vi "Get Data From Binary Block.vi"(10 "Binary Block":string) -> (2 "Data Part":string)   [LabVIEW 2016, in "Agilent 3352X Series.lvlib"]
doc: "For an IEEE Binary Block of values of the format #<n><n_digits><data>, get the <data> part of it"
uses:
  Agilent 3352X Series.lvlib
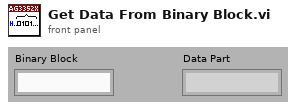
[diagram p1: front panel]
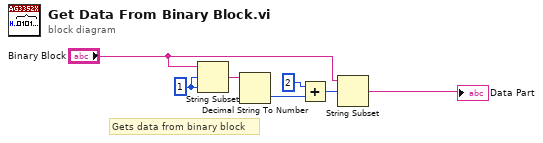
[diagram p0: block diagram]
diagram:
  w1 = 1 ("length (rest)")
  # "Gets data from binary block"
  n1 = String Subset(string="Binary Block", offset (0)=w1, length (rest)=w1) -> (substring=w7:string)
  n2 = Decimal String To Number(string=w7) -> (number=w4:i32)  [unwired: 3 out]
  n3 = Add(x=2 ("offset (0)"), y=w4) -> (x+y=w5:i32)
  n4 = String Subset(string="Binary Block", offset (0)=w5) -> (substring=→"Data Part":string)  [unwired: 1 out]
